vi "TestStep AllowAsynchronous.vi"(8 "error in (no error)":errorcluster, 11 "niDTS WLAN Rx Test in":refnum<class "niDTS WLAN Rx Test.lvclass">) -> (0 "error out":errorcluster, 2 "AllowAsynchronous":bool=TRUE, 3 "niDTS WLAN Rx Test out":refnum<class "niDTS WLAN Rx Test.lvclass">)   [LabVIEW 2015, in "niDTS WLAN.lvlib" / "niDTS WLAN Rx Test.lvclass"]
uses:
  niDTS WLAN Rx Test.lvclass
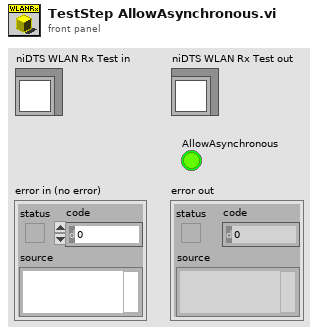
[diagram p1: front panel]
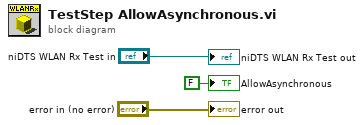
[diagram p0: block diagram]
diagram:
  "error out" <- "error in (no error)"
  "niDTS WLAN Rx Test out" <- "niDTS WLAN Rx Test in"
  "AllowAsynchronous" <- FALSE ("AllowAsynchronous")
